vi "mainFPGA.vi"() -> ()   [LabVIEW 2019]
uses:
  <vilib>/rvi/Emulation/niFpgaGetClockAttributes.vi
  <vilib>/rvi/Emulation/niFpgaSctlEmulationGetInTimedLoop.vi
  <vilib>/rvi/Emulation/niFpgaEmulationReportErrorSimple.vi
  <vilib>/rvi/eio/common/nirviEmuTemplateMethod_errors.vi
  <vilib>/rvi/Emulation/niFpgaCriticalErrorInLSC.vi
  <vilib>/eio/EIONode/EIONode.xnode
panel:
  in  "ledsControl":i32
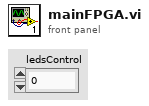
[diagram p1: front panel]
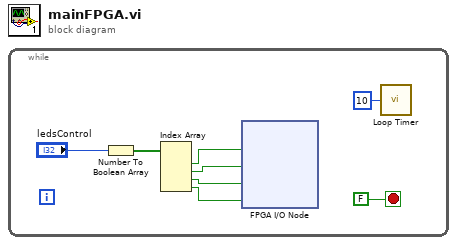
[diagram p0: block diagram]
diagram:
  n1 = while {
    stop <- FALSE stop-if-true
    n2 = Number To Boolean Array(number="ledsControl") -> (Boolean array=w8:bool[])
    n3 = Index Array(array=w8) -> (element #1=w7:bool, element #2=w6:bool, element #3=w5:bool, element #4=w3:bool)  [unwired: 4 in]
    n4 = xnode "FPGA I/O Node"("LED0"=w7, "LED1"=w6, "LED2"=w5, "LED3"=w3) -> ()  [unwired: 4 in, 4 out]
    n5 = call "Loop Timer"("Count(mSec)"=u32 10) -> ()  [unwired: 1 out]
  }
